vi "Get Result Data.vi"(8 "error in (no error)":errorcluster, 11 "Result Display in":refnum<class "Result Display.lvclass">) -> (0 "error out":errorcluster, 1 "GRR Results":T1[](array[typedef]), 2 "Test Data":T2[](array[typedef]), 3 "Result Display out":refnum<class "Result Display.lvclass">)   [LabVIEW 2018, in "Result Display.lvclass"]
uses:
  Result Display.lvclass
  TestDataMgr/Typedefs/Test Data All.ctl
  TestDataMgr/Typedefs/Test Limits.ctl
  TestDataMgr/Typedefs/Test Raw Data.ctl
  Result Data Mgr/Typedefs/GRR Result.ctl
  Result Display.lvclass/Result Display.ctl
  TestDataMgr/TestDataMgr.lvclass
  Result Data Mgr/Result Data Mgr.lvclass
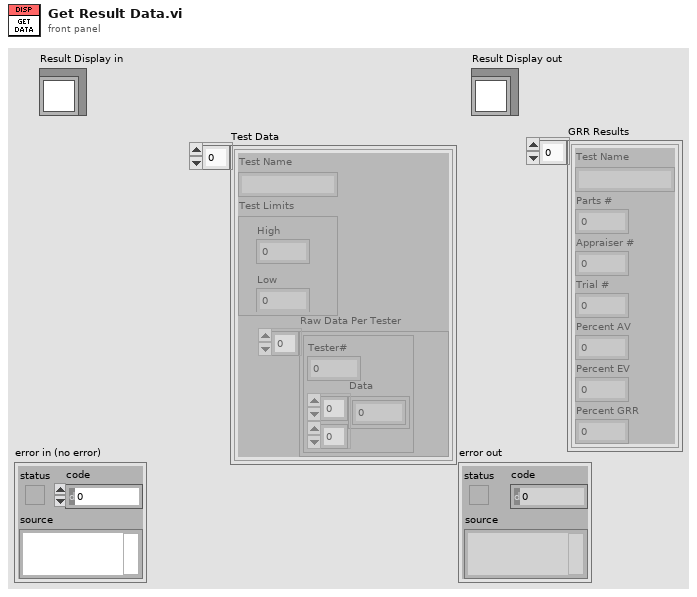
[diagram p1: front panel]
types:
  T1 = typedef "Result Data Mgr.lvclass/GRR Result.ctl" = cluster{"Test Name":string, "Parts #":u8, "Appraiser #":u8, "Trial #":u8, "Percent AV":dbl, "Percent EV":dbl, "Percent GRR":dbl}
  T2 = typedef "TestDataMgr.lvclass/Test Data All.ctl" = cluster{"Test Name":string, "Test Limits":T3, "Raw Data Per Tester":T4[]}
  T3 = typedef "TestDataMgr.lvclass/Test Limits.ctl" = cluster{"High":dbl, "Low":dbl}
  T4 = typedef "TestDataMgr.lvclass/Test Raw Data.ctl" = cluster{"Data":dbl[][], "Tester#":u8}
  T5 = typedef "TestDataMgr.lvclass/Session Handle.ctl" = refnum<data-value>
  T6 = typedef "Result Data Mgr.lvclass/Session Handle.ctl" = refnum<data-value>
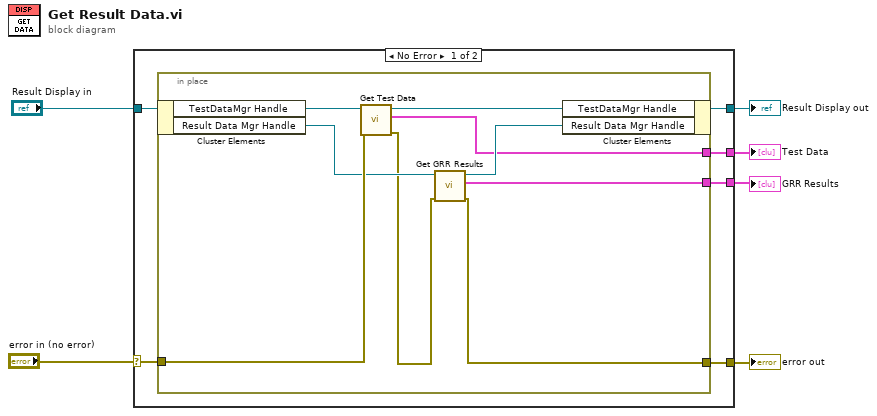
[diagram p0: block diagram]
diagram:
  n1 = case shown="No Error" "error in (no error)" {
    selector: "error in (no error)" -> [w11 w23]
    tunnel: [w9 w23] -> w5
    tunnel: [w10 w22] -> w3
    tunnel: "Result Display in" -> [w12 w22]
    tunnel: [w8 _] -> w2
    tunnel: [w7 _] -> w1
    frame No Error {
      n2 = in-place {
        in-place-border: w11 -> [w20]
        in-place-border: [w16] -> w9
        in-place-border: [w14] -> w8
        in-place-border: [w13] -> w7
        n3 = in-place-cluster #1(w12) -> ("TestDataMgr Handle"=w21:T5, "Result Data Mgr Handle"=w18:T6)
        n4 = call "Get Test Data.vi"("error in (no error)"=w20, "Session Handle in"=w21) -> ("error out"=w17:errorcluster, "Test Data"=w14:T2[], "Session Handle out"=w19:T5)  [unwired: 7 in]
        n5 = call "Get GRR Results.vi"("error in (no error)"=w17, "Session Handle in"=w18) -> ("error out"=w16:errorcluster, "GRR Results"=w13:T1[], "Session Handle out"=w15:T6)  [unwired: 7 in]
        n6 = in-place-cluster #1("TestDataMgr Handle"=w19, "Result Data Mgr Handle"=w15) -> (w10:refnum<class "Result Display.lvclass">)
      }
    }
    frame Error {
    }
  }
  "error out" <- w5
  "Result Display out" <- w3
  "Test Data" <- w2
  "GRR Results" <- w1
